vi "Konzentrationen changed.vi"(10 "TestKonfig (Eingang)":T1 {"TestKonfig Interferent"."Gasflasche MFC3" items=["----"=10000, "IAG NH3 3000"=0, "IAG NH3 200"=1, "IAG NH3 2000"=2, "IAG MG"=3, "IAG O2"=4]; "TestKonfig Interferent"."Gasflasche MFC2" items=["----"=10000, "IAG NH3 3000"=0, "IAG NH3 200"=1, "IAG NH3 2000"=2, "IAG MG"=3, "IAG O2"=4]; "TestKonfig Interferent"."Eingangs Konzentration MFC1" min=0.0; "TestKonfig Interferent"."Ausgangs Konzentration MFC1" min=0.0; "TestKonfig Interferent"."MFC2" items=["MFC 2", "MFC 3", "MFC 4", "MFC 5"]; "TestKonfig Interferent"."MFC3" items=["MFC 2", "MFC 3", "MFC 4", "MFC 5"]; "TestKonfig Interferent"."Ausgangs Konzentration MFC3" min=0.0; "TestKonfig Interferent"."Eingangs Konzentration MFC3" min=0.0; "TestKonfig Interferent"."Ausgangs Konzentration MFC2" min=0.0; "TestKonfig Interferent"."Eingangs Konzentration MFC2" min=0.0; "TestKonfig H2O"."HovaCAL Temperature" format="%.2f"; "TestKonfig H2O"."HovaCAL Flow Input Cluster"."HovaCAL Flow Input Cluster" format="%.2f"; "TestKonfig H2O"."Eingangs Konzentration:" min=0.0; "TestKonfig H2O"."zusätzliche Zeitdauer Erster Punkt" min=30 step=1 format="%#_5g"; "TestKonfig H2O"."Zeitdauer Stufen" format="%#_5g"; "TestKonfig H2O"."Max Fehler" format="%#_5g"; "TestKonfig H2O"."Anzahl Stufen" format="%#_5g"; "TestKonfig H2O"."Modus" items=["Messen", "CG zu Entnahmestelle"]}, 11 "TestKonfig alt":T1 {"TestKonfig Interferent"."Gasflasche MFC3" items=["----"=10000, "IAG NH3 3000"=0, "IAG NH3 200"=1, "IAG NH3 2000"=2, "IAG MG"=3, "IAG O2"=4]; "TestKonfig Interferent"."Gasflasche MFC2" items=["----"=10000, "IAG NH3 3000"=0, "IAG NH3 200"=1, "IAG NH3 2000"=2, "IAG MG"=3, "IAG O2"=4]; "TestKonfig Interferent"."Eingangs Konzentration MFC1" min=0.0; "TestKonfig Interferent"."Ausgangs Konzentration MFC1" min=0.0; "TestKonfig Interferent"."MFC2" items=["MFC 2", "MFC 3", "MFC 4", "MFC 5"]; "TestKonfig Interferent"."MFC3" items=["MFC 2", "MFC 3", "MFC 4", "MFC 5"]; "TestKonfig Interferent"."Ausgangs Konzentration MFC3" min=0.0; "TestKonfig Interferent"."Eingangs Konzentration MFC3" min=0.0; "TestKonfig Interferent"."Ausgangs Konzentration MFC2" min=0.0; "TestKonfig Interferent"."Eingangs Konzentration MFC2" min=0.0; "TestKonfig H2O"."HovaCAL Temperature" format="%.2f"; "TestKonfig H2O"."HovaCAL Flow Input Cluster"."HovaCAL Flow Input Cluster" format="%.2f"; "TestKonfig H2O"."Eingangs Konzentration:" min=0.0; "TestKonfig H2O"."zusätzliche Zeitdauer Erster Punkt" min=30 step=1 format="%#_5g"; "TestKonfig H2O"."Zeitdauer Stufen" format="%#_5g"; "TestKonfig H2O"."Max Fehler" format="%#_5g"; "TestKonfig H2O"."Anzahl Stufen" format="%#_5g"; "TestKonfig H2O"."Modus" items=["Messen", "CG zu Entnahmestelle"]}) -> (2 "MFC2 changed":bool, 3 "MFC3 changed":bool)   [LabVIEW 2020, in "EPA 1065.lvlib" / "HovaCAL Interference verificaton.lvlib"]
uses:
  HovaCAL Interference verificaton.lvlib
  TestKonfig.ctl
  TestKonfig H2O.ctl
  Modus.ctl
  Linearisierung V2/SpanEinstellungen/Einheit.ctl
  Linearisierung V2/Gasteiler/Stufen Tabelle 10 Stufen.ctl
  Linearisierung V2/Gasteiler/HovaCAL_Interface/Controls/Flow Einstellung.ctl
  Linearisierung V2/Gasteiler/HovaCAL_Interface/Controls/Temp Sollwerte Anzeige.ctl
  TestKonfig Interferents.ctl
  MFCAuswahl.ctl
  Seiten/System Einstellungen V2/Gasflasche Auswahl.ctl
  Linearisierung V2/SpanEinstellungen/SpanEinstellungen.lvlib
  Linearisierung V2/Gasteiler/Gasteiler.lvlib
  Linearisierung V2/Gasteiler/HovaCAL_Interface/Controls/Controls.lvlib
  Seiten/System Einstellungen V2/System Einstellungen V2.lvlib
panel:
  # "sec"
  # "%"
  # "sec"
  # "sec"
  # "%"
  # "sec"
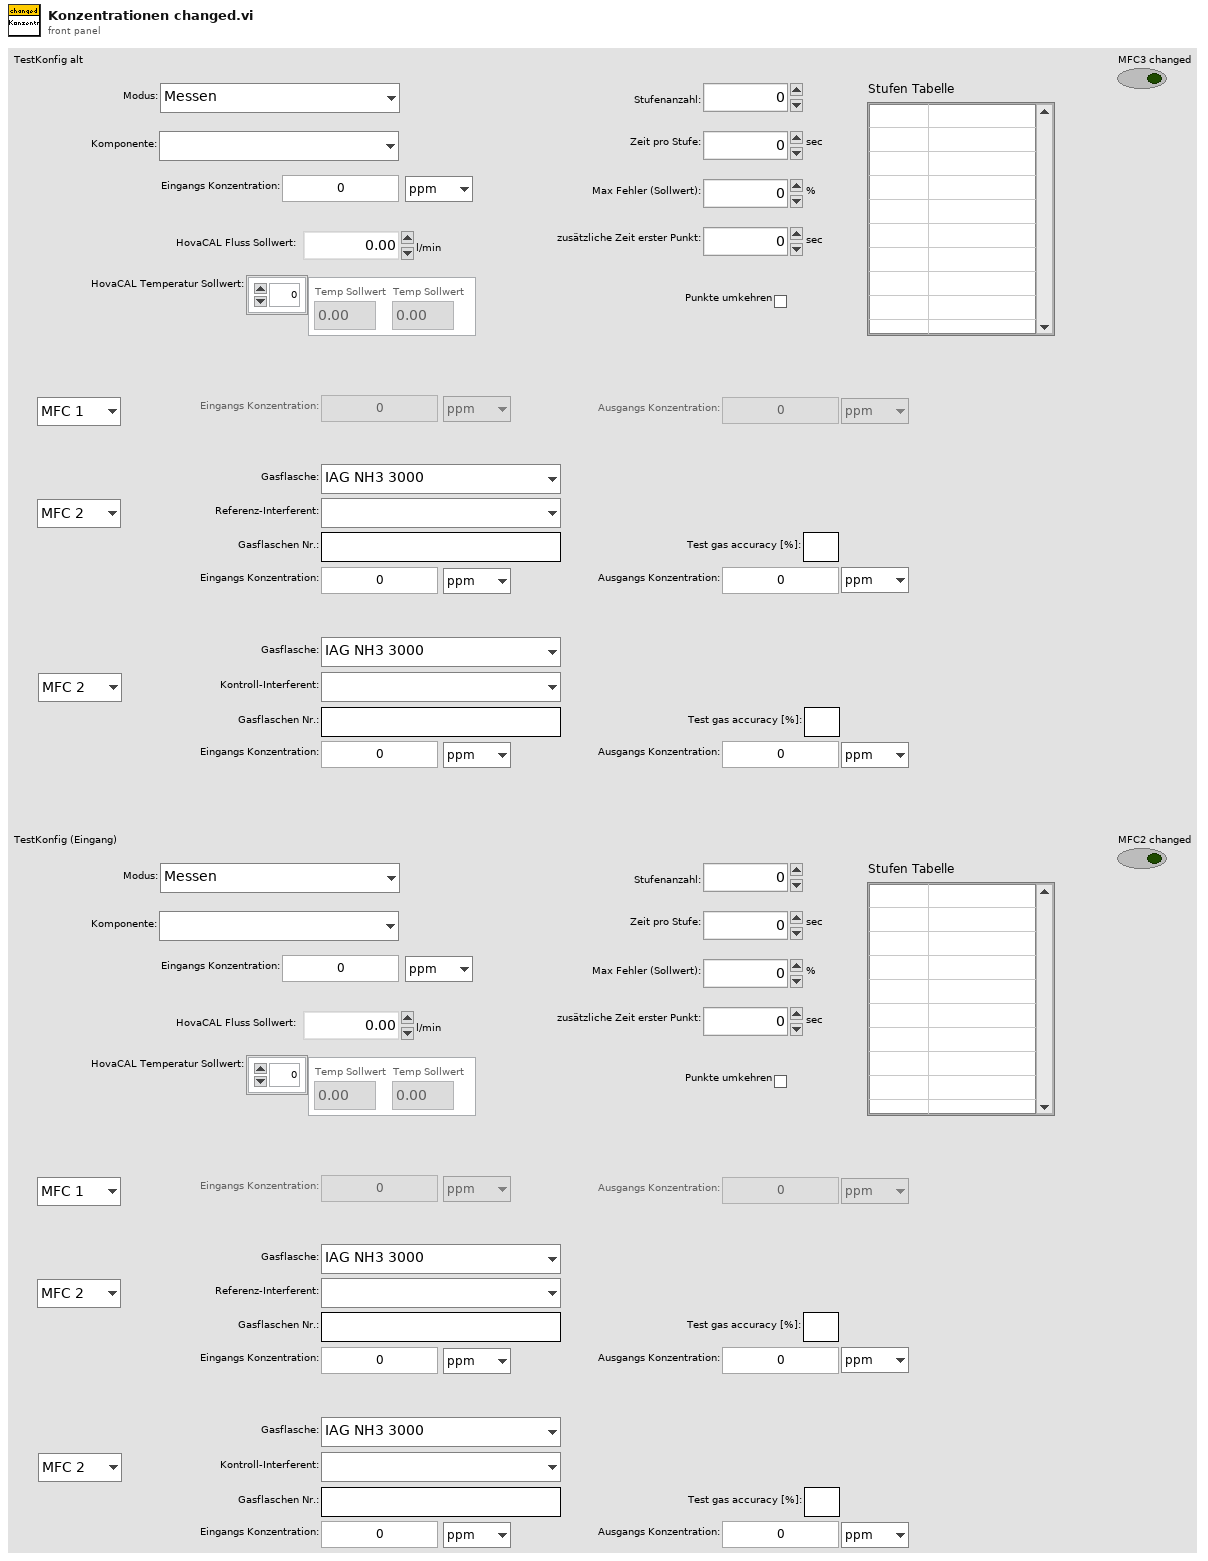
[diagram p1: front panel]
types:
  T1 = typedef "EPA 1065.lvlib/HovaCAL Interference verificaton.lvlib/TestKonfig.ctl" = cluster{"TestKonfig H2O":T2, "TestKonfig Interferent":T8}
  T2 = typedef "EPA 1065.lvlib/HovaCAL Interference verificaton.lvlib/TestKonfig H2O.ctl" = cluster{"Modus":T3, "Komponente:":u16, "Eingangs Konzentration:":dbl, "Einheit":T4, "Anzahl Stufen":sgl, "Zeitdauer Stufen":sgl, "Max Fehler":sgl, "zusätzliche Zeitdauer Erster Punkt":sgl, "Punkte umkehren":bool, "Stufen Tabelle":T5, "HovaCAL Flow Input Cluster":T6, "HovaCAL Temperature":T7}
  T3 = typedef "EPA 1065.lvlib/HovaCAL Interference verificaton.lvlib/Modus.ctl" = u16
  T4 = typedef "Linearisierung v2.lvlib/SpanEinstellungen.lvlib/Einheit.ctl" = enum16{"ppm", "%"}
  T5 = typedef "Linearisierung v2.lvlib/Gasteiler.lvlib/Stufen Tabelle 10 Stufen.ctl" = string[][]
  T6 = typedef "Linearisierung v2.lvlib/Gasteiler.lvlib/HovaCAL_Interface.lvlib/Controls.lvlib/Flow Einstellung.ctl" = cluster{"HovaCAL Flow Input Cluster":dbl}
  T7 = typedef "Linearisierung v2.lvlib/Gasteiler.lvlib/HovaCAL_Interface.lvlib/Controls.lvlib/Temp Sollwerte Anzeige.ctl" = dbl[]
  T8 = typedef "EPA 1065.lvlib/HovaCAL Interference verificaton.lvlib/TestKonfig Interferents.ctl" = cluster{"MFC1":enum16{"MFC 1"}, "Eingangs Konzentration MFC1":dbl, "Einheit MFC1 Eingang":T4, "Ausgangs Konzentration MFC1":dbl, "Einheit MFC1 Ausgang":T4, "MFC2":T9, "Referenz-Interferent:":u16, "Gasflaschen Nr MFC2":string, "Accuracy MFC2":string, "Eingangs Konzentration MFC2":dbl, "Einheit MFC2 Eingang":T4, "Ausgangs Konzentration MFC2":dbl, "Einheit MFC2 Ausgang":T4, "MFC3":T9, "Kontroll-Interferent:":u16, "Gasflaschen Nr MFC3":string, "Accuracy MFC3":string, "Eingangs Konzentration MFC3":dbl, "Einheit MFC3 Eingang":T4, "Ausgangs Konzentration MFC3":dbl, "Einheit MFC3 Ausgang":T4, "Gasflasche MFC2":T10, "Gasflasche MFC3":T10}
  T9 = typedef "EPA 1065.lvlib/HovaCAL Interference verificaton.lvlib/MFCAuswahl.ctl" = u16
  T10 = typedef "System Einstellungen V2.lvlib/Gasflasche Auswahl.ctl" = u16
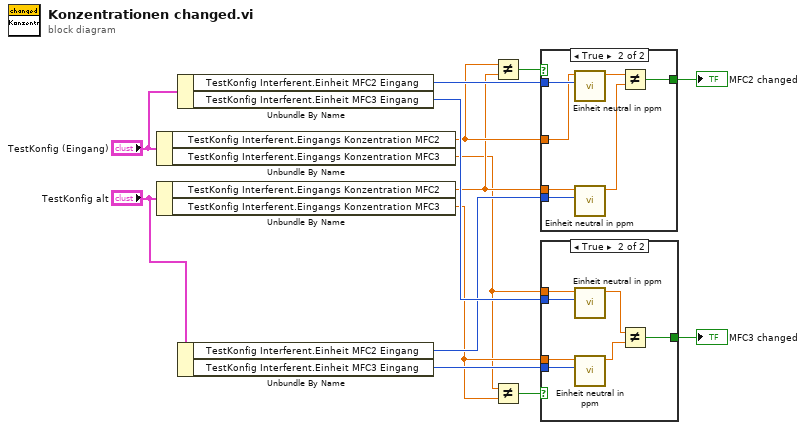
[diagram p0: block diagram]
diagram:
  n1 = Unbundle By Name("TestKonfig (Eingang)") -> ("TestKonfig Interferent.Eingangs Konzentration MFC2"=w6:dbl, "TestKonfig Interferent.Eingangs Konzentration MFC3"=w2:dbl)
  n2 = Unbundle By Name("TestKonfig alt") -> ("TestKonfig Interferent.Eingangs Konzentration MFC2"=w5:dbl, "TestKonfig Interferent.Eingangs Konzentration MFC3"=w3:dbl)
  n3 = Unbundle By Name("TestKonfig (Eingang)") -> ("TestKonfig Interferent.Einheit MFC2 Eingang"=w12:T4, "TestKonfig Interferent.Einheit MFC3 Eingang"=w11:T4)
  n4 = Unbundle By Name("TestKonfig alt") -> ("TestKonfig Interferent.Einheit MFC2 Eingang"=w10:T4, "TestKonfig Interferent.Einheit MFC3 Eingang"=w7:T4)
  n5 = Not Equal?(x=w6, y=w5) -> (x != y?=w4:bool)
  n6 = Not Equal?(x=w2, y=w3) -> (x != y?=w1:bool)
  n7 = case shown="True" w4 {
    tunnel: [_ w21] -> w14
    tunnel: w12 -> [_ w20]
    tunnel: w10 -> [_ w17]
    tunnel: w6 -> [_ w16]
    tunnel: w5 -> [_ w15]
    frame False {
    }
    frame True {
      n8 = call "Einheit neutral in ppm.vi"("Einheit"=w20, "Konzentration in"=w16) -> ("Konzentration out"=w19:dbl)  [unwired: 9 in]
      n9 = call "Einheit neutral in ppm.vi"("Einheit"=w17, "Konzentration in"=w15) -> ("Konzentration out"=w18:dbl)  [unwired: 9 in]
      n10 = Not Equal?(x=w19, y=w18) -> (x != y?=w21:bool)
    }
  }
  "MFC2 changed" <- w14
  n11 = case shown="True" w1 {
    tunnel: [_ w28] -> w13
    tunnel: w2 -> [_ w27]
    tunnel: w11 -> [_ w26]
    tunnel: w3 -> [_ w24]
    tunnel: w7 -> [_ w22]
    frame False {
    }
    frame True {
      n12 = call "Einheit neutral in ppm.vi"("Einheit"=w26, "Konzentration in"=w27) -> ("Konzentration out"=w25:dbl)  [unwired: 9 in]
      n13 = call "Einheit neutral in ppm.vi"("Einheit"=w22, "Konzentration in"=w24) -> ("Konzentration out"=w23:dbl)  [unwired: 9 in]
      n14 = Not Equal?(x=w25, y=w23) -> (x != y?=w28:bool)
    }
  }
  "MFC3 changed" <- w13
